vi "GUI_Plasma2_GasJetInterferometry.vi"() -> ()   [LabVIEW 2020]
uses:
  Shared/GUI_Template/GUI_master/tcp_new_data_event.ctl
  Shared/GUI_Template/GUI_master/tcp new data cluster.ctl
  Device Drivers/DG645/subVIs/TriggerSource_TypDef.ctl
panel:
  in  "Trigger.Rate::1":dbl=0.3 caption="Rate (Hz)" min=0.001 max=1000.0
  in  "Trigger.Source::1":T1 caption="SRS Trigger Mode"
  in  "Pressure.device 1::2":dbl caption="pressure (psi)" min=0.0 max=500.0 format="%.3f"
  in  "Delay.Ch B::1":dbl caption="open time" min=-0.1 max=0.1 format="%.3p"
  in  "Delay.Ch A::1":dbl caption="jet delay" min=-0.1 max=0.1 format="%.3p"
  in  "GUIdevice 2":string="PRC-P2-Alicat"
  in  "GUIdevice 1":string="P2FastDiag645"
  in  "stop":bool
  out "tcp data event":T2
  out "error IO 2":errorcluster
  # "PL2 CONTROL CENTER"
  # "Jet"
  # "DG"
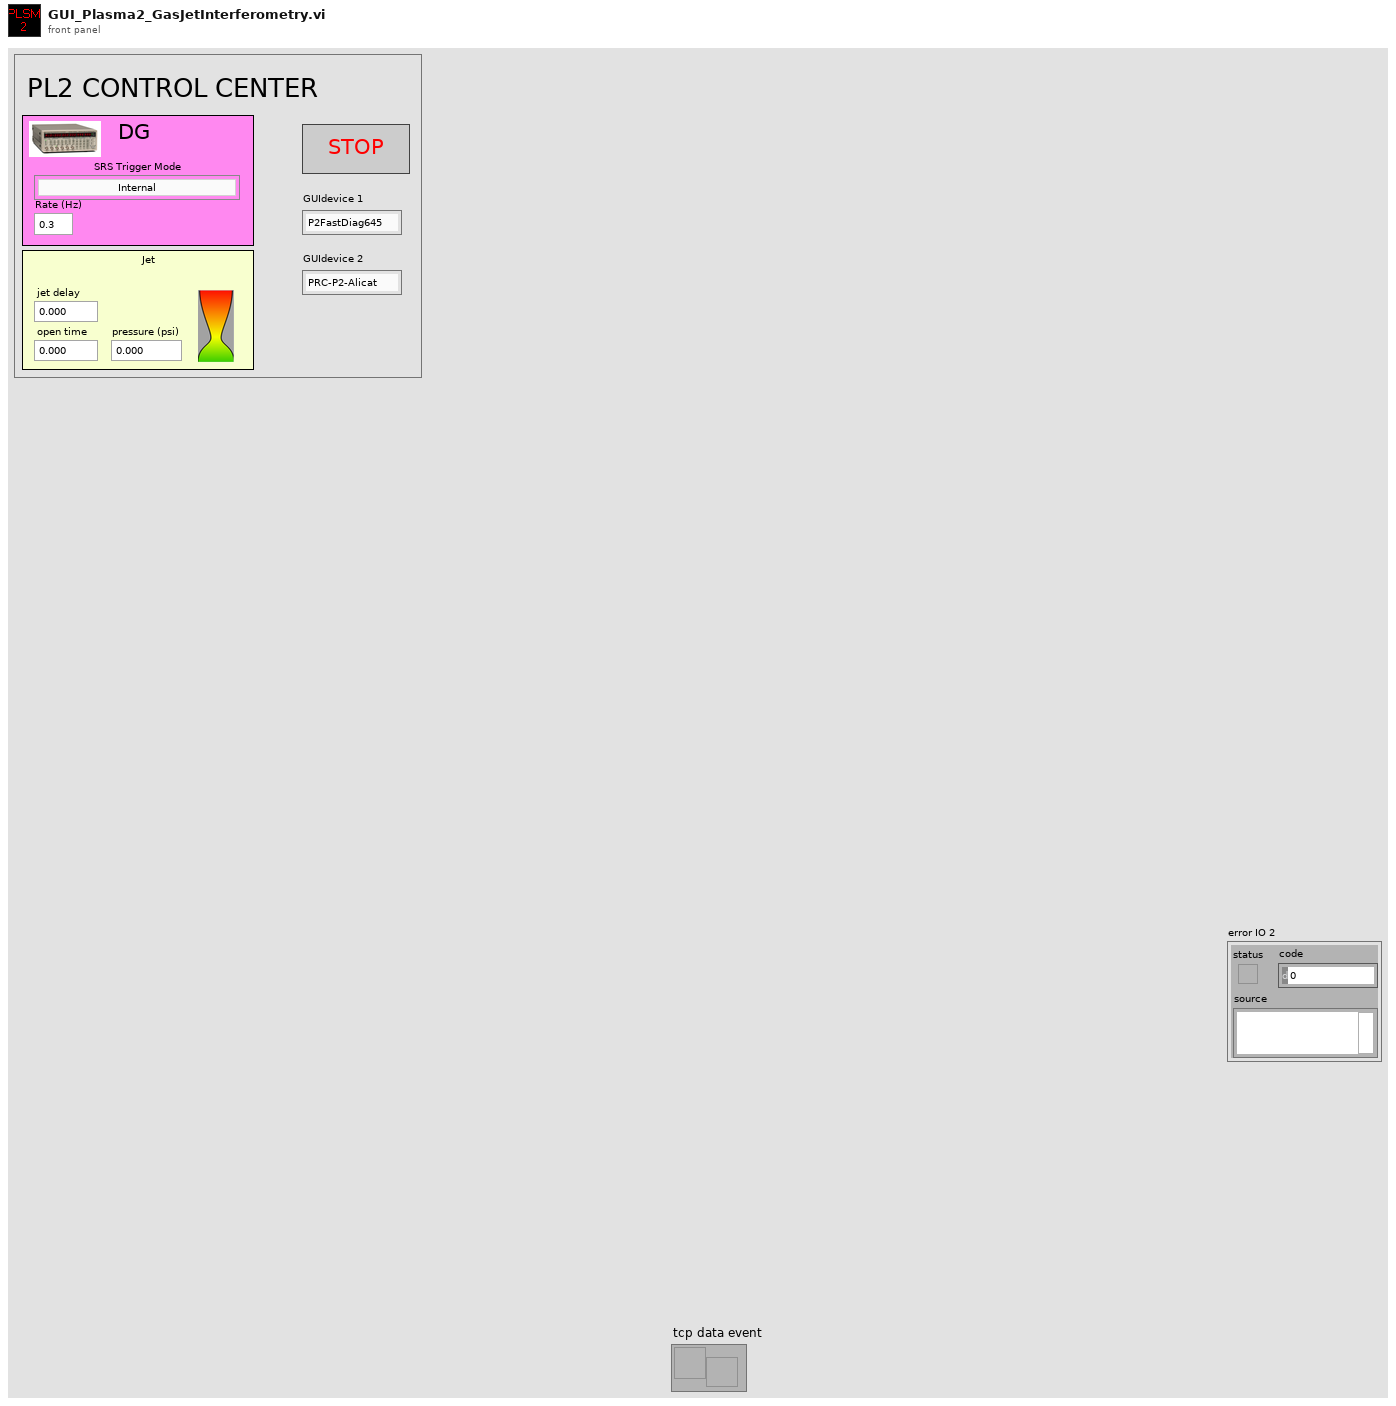
[diagram p1: front panel]
types:
  T1 = typedef "TriggerSource_TypDef.ctl" = enum16{"Internal", "External rising edges", "External falling edges", "Single shot external rising edges", "Single shot external falling edges", "Single shot", "Line"}
  T2 = typedef "tcp_new_data_event.ctl" = refnum<user-event>
  T3 = typedef "tcp new data cluster.ctl" = cluster{"EventEnum":enum16{"new data", "connection status update"}, "Device name":string}
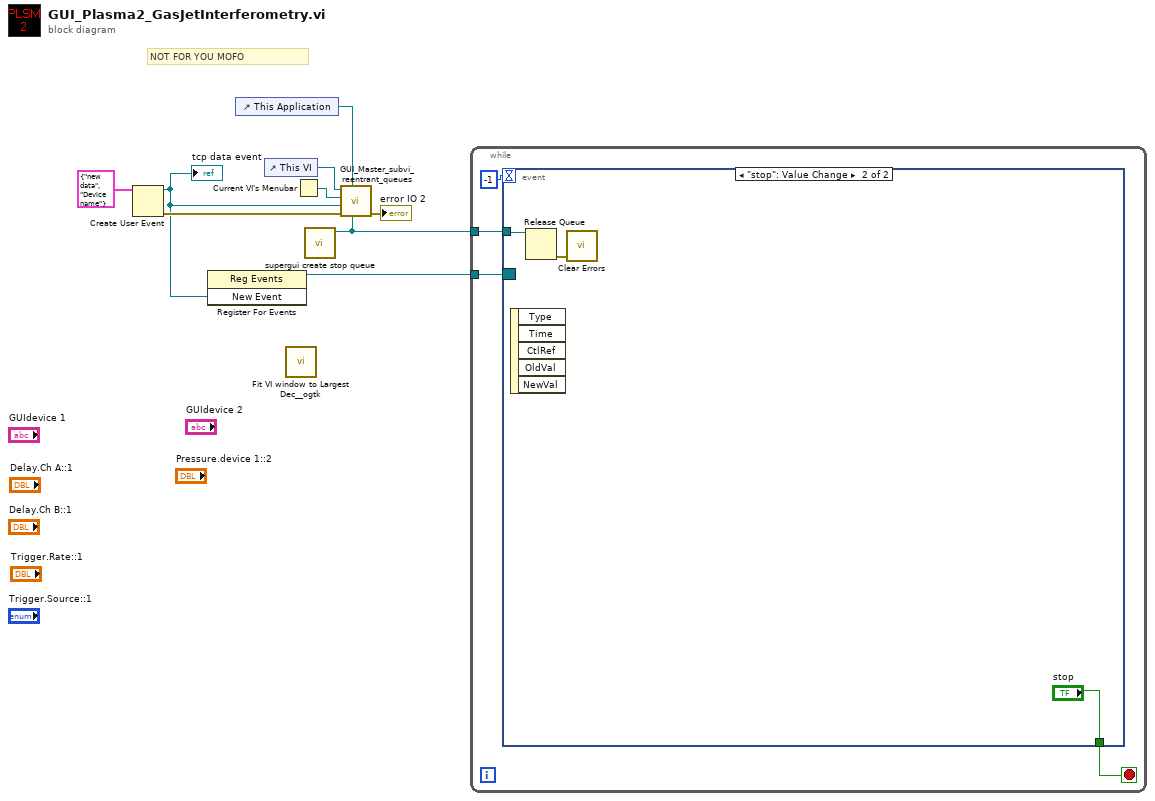
[diagram p0: block diagram]
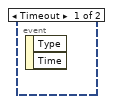
[diagram p2: hidden frame]
diagram:
  # "NOT FOR YOU MOFO"
  n1 = Create User Event(user event datatype=T3 {"EventEnum"=enum."new data", "Device name"="Device name"} ("New Event")) -> (user event=w4:refnum<user-event>, error out=w5:errorcluster)  [unwired: 1 in]
  "tcp data event" <- w4
  n2 = register-events(w4) -> (reference out=w2:refnum<event-registration>)  [unwired: 2 in, 1 out]
  n3 = control-ref of="This Application"() -> (w3:refnum<vi>)
  n4 = control-ref of="This VI"() -> (w8:refnum<vi>)
  n5 = call <userlib>:"Fit VI window to Largest Dec__ogtk.vi"() -> ()  [unwired: 6 in, 2 out]
  n6 = Current VI's Menubar() -> (w7:refnum<k9>)
  n7 = call "supergui create stop queue.vi"() -> ("STOP Queue out"=w1:refnum<queue>)  [unwired: 11 in]
  n8 = call "GUI_Master_subvi_reentrant_queues.vi"("STOP Queue in"=w1, "This Application"=w3, "error in (no error)"=w5, "tcp data event"=w4, "Caller menu reference"=w7, "Caller VI ref"=w8) -> ("error out"=→"error IO 2":errorcluster)  [unwired: 5 in]
  n9 = while {
    tunnel: w2 -> [w12]
    tunnel: w1 -> [w10]
    stop <- w13 stop-if-true
    n10 = event shown="[1] \"stop\": Value Change" {
      selector: w12 -> [_ _]
      dyn-events: _ -> [_ _]
      timeout: -1 -> [_ _]
      tunnel: [_ "stop"] -> w13
      tunnel: w10 -> [_ w14]
      event Timeout {
        n11 = event-data() -> ()  [unwired: 1 in, 2 out]
      }
      event "stop": Value Change {
        n12 = event-data() -> ()  [unwired: 1 in, 5 out]
        n13 = Release Queue(queue=w14) -> (error out=w15:errorcluster)  [unwired: 2 in, 2 out]
        n14 = call <vilib>:"Clear Errors.vi"("error in (no error)"=w15) -> ()  [unwired: 5 in, 2 out]
      }
    }
  }
